vi "StringToPythonBuffer.vi"(5 "Buffer":bool=TRUE, 8 "string":string) -> (2 "python string":string)   [LabVIEW 2014, in "Raspberry Pi Compatible Compiler for LabVIEW.lvlib" / "Python Functions.lvlib"]
uses:
  Python Functions.lvlib
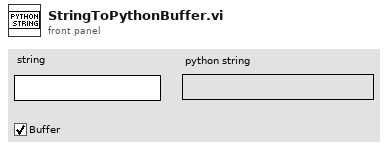
[diagram p1: front panel]
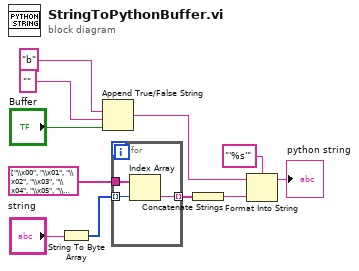
[diagram p0: block diagram]
diagram:
  n1 = String To Byte Array(string="string") -> (unsigned byte array=w6:u8[])
  n2 = Append True/False String(1:"Buffer", 2:"" ("false string"), 3:"b" ("true string")) -> (0:w2:string)  [unwired: 1 in]
  n3 = for {
    tunnel: string[] ["\\x00", "\\x01", "\\x02", "\\x03", "\\x04", "\\x05", "\\x06", "\\x07", "\\x08", "\\x09", "\\x0A", "\\x0B", "\\x0C", "\\x0D", "\\x0E", "\\x0F", "\\x10", "\\x11", "\\x12", "\\x13", "\\x14", "\\x15", "\\x16", "\\x17", "\\x18", "\\x19", "\\x1A", "\\x1B", "\\x1C", "\\x1D", "\\x1E", "\\x1F", "\\x20", "!", "\\\"", "#", "$", "%", "&", "\\'", "(", ")", "*", "+", ",", "-", ".", "/", "0", "1", "2", "3", "4", "5", "6", "7", "8", "9", ":", ";", "<", "=", ">", "?", "@", "A", "B", "C", "D", "E", "F", "G", "H", "I", "J", "K", "L", "M", "N", "O", "P", "Q", "R", "S", "T", "U", "V", "W", "X", "Y", "Z", "[", "\\", "]", "^", "_", "`", "a", "b", "c", "d", "e", "f", "g", "h", "i", "j", "k", "l", "m", "n", "o", "p", "q", "r", "s", "t", "u", "v", "w", "x", "y", "z", "{", "|", "}", "~", "\\x7F", "\\x80", "\\x81", "\\x82", "\\x83", "\\x84", "\\x85", "\\x86", "\\x87", "\\x88", "\\x89", "\\x8A", "\\x8B", "\\x8C", "\\x8D", "\\x8E", "\\x8F", "\\x90", "\\x91", "\\x92", "\\x93", "\\x94", "\\x95", "\\x96", "\\x97", "\\x98", "\\x99", "\\x9A", "\\x9B", "\\x9C", "\\x9D", "\\x9E", "\\x9F", "\\xA0", "\\xA1", "\\xA2", "\\xA3", "\\xA4", "\\xA5", "\\xA6", "\\xA7", "\\xA8", "\\xA9", "\\xAA", "\\xAB", "\\xAC", "\\xAD", "\\xAE", "\\xAF", "\\xB0", "\\xB1", "\\xB2", "\\xB3", "\\xB4", "\\xB5", "\\xB6", "\\xB7", "\\xB8", "\\xB9", "\\xBA", "\\xBB", "\\xBC", "\\xBD", "\\xBE", "\\xBF", "\\xC0", "\\xC1", "\\xC2", "\\xC3", "\\xC4", "\\xC5", "\\xC6", "\\xC7", "\\xC8", "\\xC9", "\\xCA", "\\xCB", "\\xCC", "\\xCD", "\\xCE", "\\xCF", "\\xD0", "\\xD1", "\\xD2", "\\xD3", "\\xD4", "\\xD5", "\\xD6", "\\xD7", "\\xD8", "\\xD9", "\\xDA", "\\xDB", "\\xDC", "\\xDD", "\\xDE", "\\xDF", "\\xE0", "\\xE1", "\\xE2", "\\xE3", "\\xE4", "\\xE5", "\\xE6", "\\xE7", "\\xE8", "\\xE9", "\\xEA", "\\xEB", "\\xEC", "\\xED", "\\xEE", "\\xEF", "\\xF0", "\\xF1", "\\xF2", "\\xF3", "\\xF4", "\\xF5", "\\xF6", "\\xF7", "\\xF8", "\\xF9", "\\xFA", "\\xFB", "\\xFC", "\\xFD", "\\xFE", "\\xFF"] ("Array") -> [w13]
    tunnel: w6 -> [w14] mode=indexing
    tunnel: [w12] -> w5 mode=indexing
    n4 = Index Array(array=w13, index=w14) -> (element=w12:string)
  }
  n5 = Concatenate Strings(w5) -> (w10:string)
  n6 = Format Into String(format string="'%s'", initial string=w2, w10) -> (resulting string=→"python string":string)  [unwired: 1 in, 1 out]
